vi "Configure Head and Air.vi"(8 "error in (no error)":errorcluster, 10 "Head and Air actions":T1, 11 "Temperature Control in":refnum<class "Temperature Control.lvclass">) -> (0 "error out":errorcluster, 3 "Temperature Control out":refnum<class "Temperature Control.lvclass">)   [LabVIEW 2020, in "Temperature Control.lvclass"]
doc: "Configures the Head position, Air flow and compressor."
uses:
  Temperature Control.lvclass
  Controls/Head and Air actions.ctl
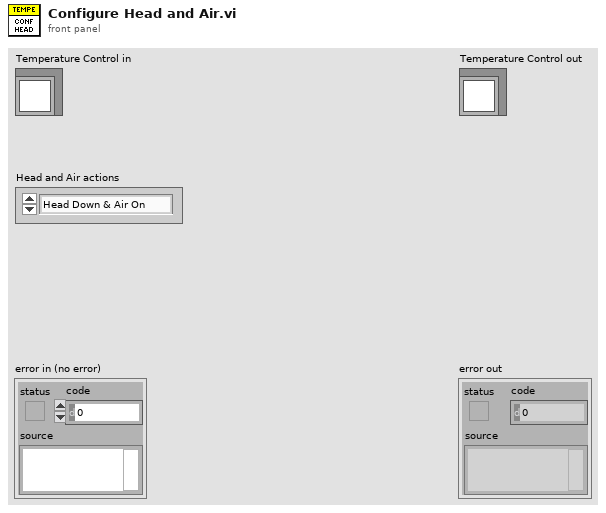
[diagram p1: front panel]
types:
  T1 = typedef "Temperature Control.lvclass/Head and Air actions.ctl" = enum16{"Head Down & Air On", "Head Up & Air Off", "Head Down", "Head Up", "Air On", "Air Off", "Compressor On", "Compressor Off"}
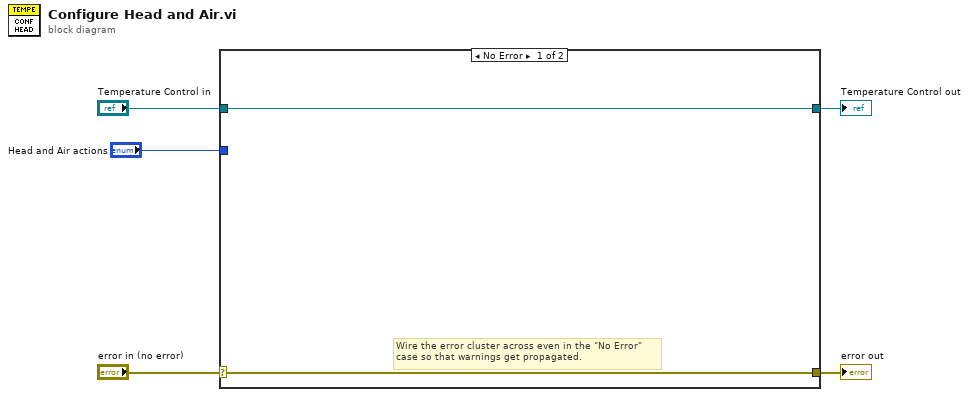
[diagram p0: block diagram]
diagram:
  n1 = case shown="No Error" "error in (no error)" {
    selector: "error in (no error)" -> [w6 w9]
    tunnel: [w6 w9] -> w4
    tunnel: [w7 w8] -> w2
    tunnel: "Temperature Control in" -> [w7 w8]
    tunnel: "Head and Air actions" -> [_ _]
    frame No Error {
      # "Wire the error cluster across even in the \"No Error\"\ncase so that warnings get propagated."
    }
    frame Error {
    }
  }
  "error out" <- w4
  "Temperature Control out" <- w2
